vi "Start Countdown.vi"(8 "error in (no error)":errorcluster, 10 "Step Length":dbl, 11 "Simulated Wash Display Console in":refnum<class "Simulated Wash Display Console.lvclass">) -> (0 "error out":errorcluster, 3 "Simulated Wash Display Console out":refnum<class "Simulated Wash Display Console.lvclass">)   [LabVIEW 2012, in "Simulated Wash Display Console.lvlib" / "Simulated Wash Display Console.lvclass"]
uses:
  Simulated Wash Display Console.lvclass
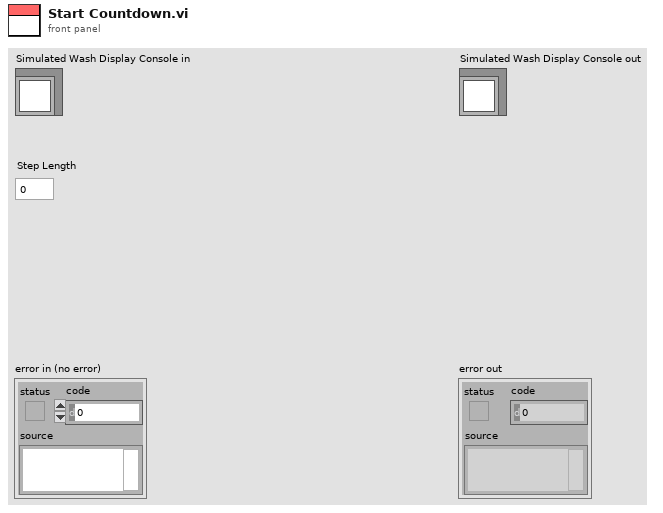
[diagram p1: front panel]
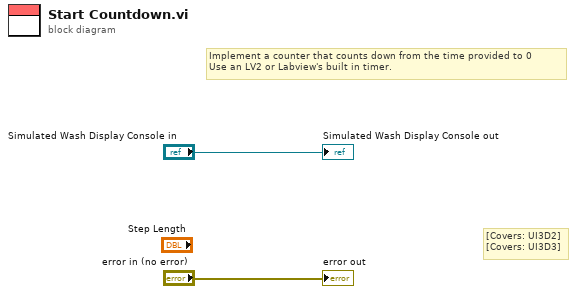
[diagram p0: block diagram]
diagram:
  # "[Covers: UI3D2]\n[Covers: UI3D3]"
  # "Implement a counter that counts down from the time provided to 0\nUse an LV2 or Labview's built in timer."
  "error out" <- "error in (no error)"
  "Simulated Wash Display Console out" <- "Simulated Wash Display Console in"
